vi "0816147.vi"() -> ()   [LabVIEW 2021]
uses:
  <vilib>/gmath/NI_Gmath.lvlib
panel:
  in  "OFF以外的按鍵":T1
  out "七段顯示器小數點":bool
  out "七段顯示器是+ or -":string
  out "七段顯示器":u16[](array[ring])
  out "七段顯示器的=":string
  out "y value 2":dbl format="%.2f"
  in  "formula":string
  out "目前時間":timestamp format="%<%X\n%x>T"
  out "計算機已執行時間":string
  in  "off":bool
  out "算式顯示":string caption="String"
  out "答案":dbl
  in  "計算機背景圖片":u16(ring)
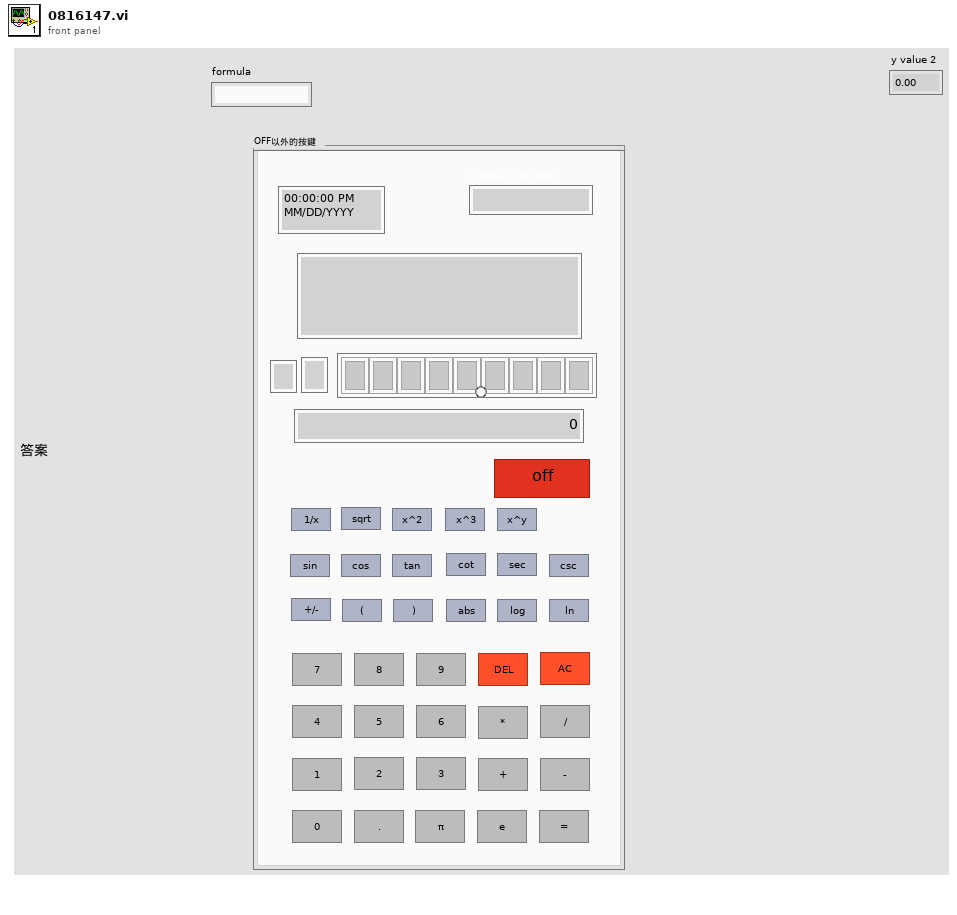
[diagram p1: front panel]
types:
  T1 = cluster{"0":bool, "1":bool, "2":bool, "3":bool, "4":bool, "5":bool, "6":bool, "7":bool, "8":bool, "9":bool, ".":bool, "pi":bool, "e":bool, "/":bool, "*":bool, "-":bool, "=":bool, "DEL":bool, "+":bool, "cos":bool, "sin":bool, "(":bool, ")":bool, "tan":bool, "log":bool, "ln":bool, "x^2":bool, "sqrt":bool, "x^3":bool, "AC":bool, "+/-":bool, "x^y":bool, "csc":bool, "sec":bool, "cot":bool, "1/x":bool, "abs":bool}
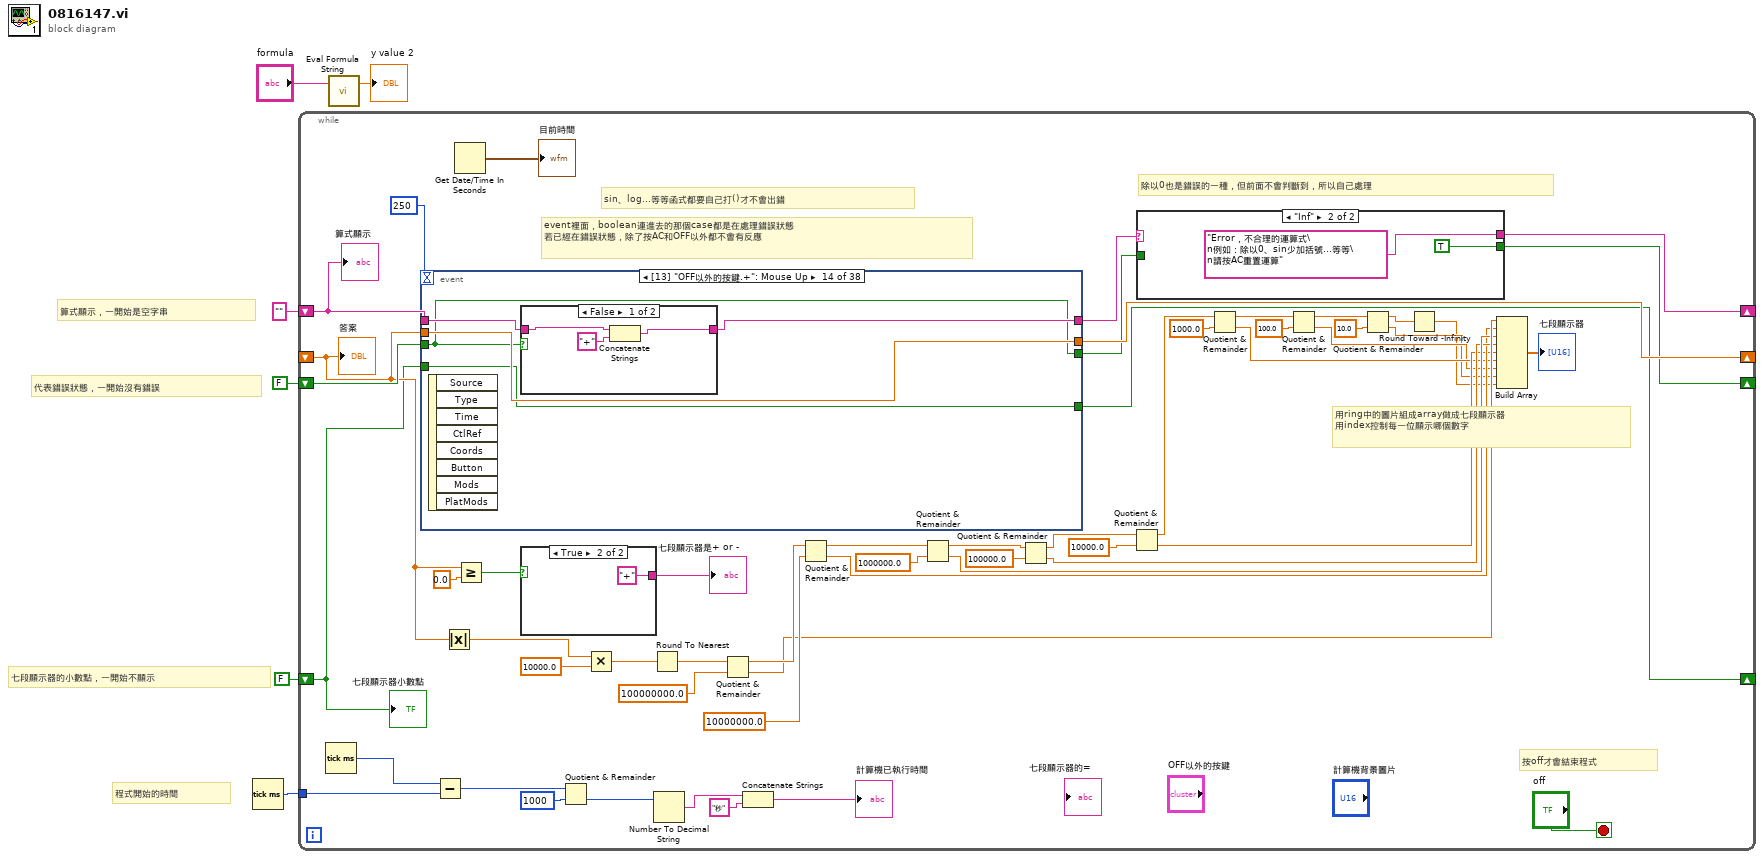
[diagram p0: block diagram]
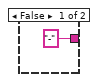
[diagram p2: hidden frame]
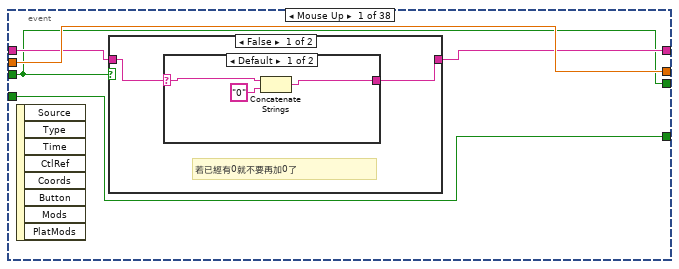
[diagram p4: hidden frame]
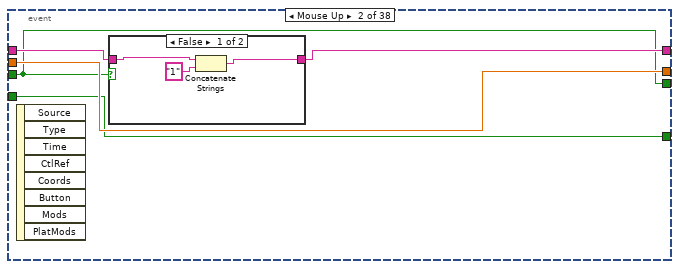
[diagram p7: hidden frame]
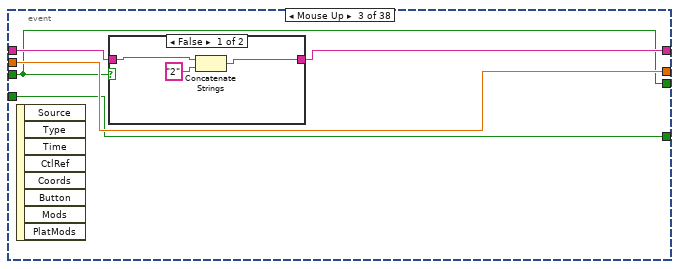
[diagram p9: hidden frame]
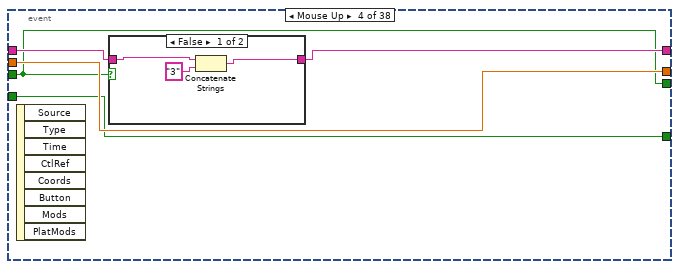
[diagram p11: hidden frame]
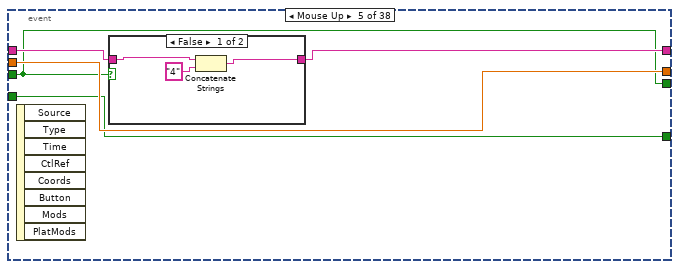
[diagram p13: hidden frame]
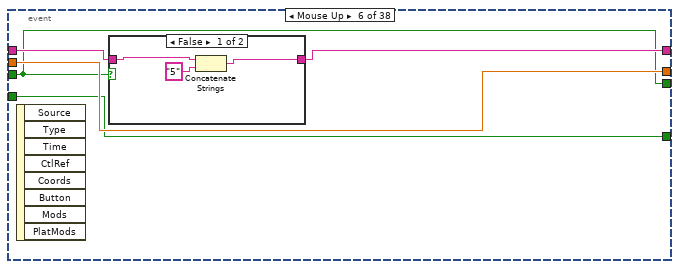
[diagram p15: hidden frame]
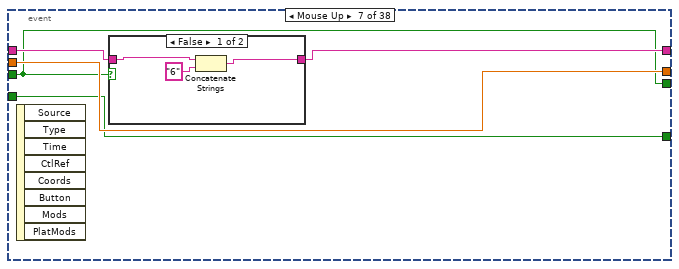
[diagram p17: hidden frame]
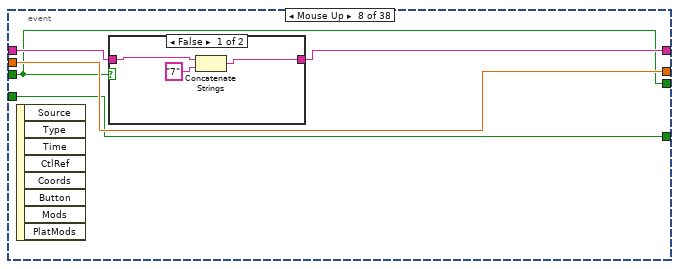
[diagram p19: hidden frame]
diagram:
  # "程式開始的時間"
  # "七段顯示器的小數點，一開始不顯示"
  # "代表錯誤狀態，一開始沒有錯誤"
  # "算式顯示，一開始是空字串"
  n1 = Tick Count (ms)() -> (millisecond timer value=w5:u32)
  n2 = while {
    shift-right: [w44] -> _
    shift-left: "" -> [w43]
    tunnel: w5 -> [w58]
    shift-right: [w50] -> _
    shift-left: _ -> [w39]
    shift-right: [w45] -> _
    shift-left: FALSE -> [w48]
    shift-right: [w20] -> _
    shift-left: FALSE -> [w19]
    stop <- "off" stop-if-true
    # "sin、log...等等函式都要自己打()才不會出錯"
    # "按off才會結束程式"
    # "除以0也是錯誤的一種，但前面不會判斷到，所以自己處理"
    # "用ring中的圖片組成array做成七段顯示器\n用index控制每一位顯示哪個數字"
    # "event裡面，boolean連進去的那個case都是在處理錯誤狀態\n若已經在錯誤狀態，除了按AC和OFF以外都不會有反應"
    n3 = Tick Count (ms)() -> (millisecond timer value=w60:u32)
    n4 = event shown="[13] \"OFF以外的按鍵.+\": Mouse Up" {
      selector: _ -> [_ _ _ _ _ _ _ _ _ _ _ _ _ _ _ _ _ _ _ _ _ _ _ _ _ _ _ _ _ _ _ _ _ _ _ _ _ _]
      dyn-events: _ -> [_ _ _ _ _ _ _ _ _ _ _ _ _ _ _ _ _ _ _ _ _ _ _ _ _ _ _ _ _ _ _ _ _ _ _ _ _ _]
      timeout: 250 -> [_ _ _ _ _ _ _ _ _ _ _ _ _ _ _ _ _ _ _ _ _ _ _ _ _ _ _ _ _ _ _ _ _ _ _ _ _ _]
      tunnel: w43 -> [w70 w82 w91 w100 w109 w118 w127 w136 w144 w153 w162 w172 w183 w197 w206 w215 w224 w230 w247 w264 w273 w282 w291 w300 w309 w319 w328 w336 w345 w354 w363 w372 w382 w389 w400 w408 w417 w432]
      tunnel: [w69 w81 w90 w99 w108 w117 w126 w135 w143 w152 w161 w171 w182 w196 w205 w214 w223 w236 w246 w263 w272 w281 w290 w299 w308 w318 w327 w335 w344 w353 w362 w371 w381 w388 w397 w407 w422 w432] -> w47
      tunnel: [w71 w83 w92 w101 w110 w119 w128 w137 w146 w155 w164 w174 w184 w198 w207 w216 w225 w238 w244 w265 w274 w283 w292 w301 w310 w317 w326 w337 w346 w355 w364 w373 w380 w390 w399 w409 w421 w431] -> w50
      tunnel: w39 -> [w71 w83 w92 w101 w110 w119 w128 w137 w146 w155 w164 w174 w184 w198 w207 w216 w225 _ w244 w265 w274 w283 w292 w301 w310 w317 w326 w337 w346 w355 w364 w373 w380 w390 w399 w409 w416 w431]
      tunnel: [w68 w80 w89 w98 w107 w116 w125 w134 w145 w154 w163 w173 w181 w195 w204 w213 w222 w234 w245 w262 w271 w280 w289 w298 w307 w316 w325 w334 w343 w352 w361 w370 w379 w391 w398 w406 w420 w430] -> w46
      tunnel: w48 -> [w68 w80 w89 w98 w107 w116 w125 w134 w145 w154 w163 w173 w181 w195 w204 w213 w222 _ w245 w262 w271 w280 w289 w298 w307 w316 w325 w334 w343 w352 w361 w370 w379 w391 w398 w406 w418 w430]
      tunnel: [w67 w79 w88 w97 w106 w115 w124 w133 w142 w151 w160 w170 w180 w194 w203 w212 w221 w231 w243 w261 w270 w279 w288 w297 w306 w315 w324 w333 w342 w351 w360 w369 w378 w387 w396 w405 w415 w429] -> w20
      tunnel: w19 -> [w67 w79 w88 w97 w106 w115 w124 w133 w142 w151 w160 w170 w180 w194 w203 w212 w221 _ w243 w261 w270 w279 w288 w297 w306 w315 w324 w333 w342 w351 w360 w369 w378 w387 w396 w405 w415 w429]
      event "OFF以外的按鍵.0": Mouse Up {
        n5 = event-data() -> ()  [unwired: 1 in, 8 out]
        n6 = case shown="False" w68 {
          tunnel: w70 -> [w73 w78]
          tunnel: [w72 w78] -> w69
          frame False {
            # "若已經有0就不要再加0了"
            n7 = case shown="Default" w73 {
              selector: w73 -> [w75 w77]
              tunnel: [w74 w77] -> w72
              frame Default {
                n8 = Concatenate Strings(w75, "0") -> (w74:string)
              }
              frame "0" {
              }
            }
          }
          frame True {
          }
        }
      }
      event "OFF以外的按鍵.1": Mouse Up {
        n9 = event-data() -> ()  [unwired: 1 in, 8 out]
        n10 = case shown="False" w80 {
          tunnel: w82 -> [w86 w87]
          tunnel: [w84 w87] -> w81
          frame False {
            n11 = Concatenate Strings(w86, "1") -> (w84:string)
          }
          frame True {
          }
        }
      }
      event "OFF以外的按鍵.2": Mouse Up {
        n12 = event-data() -> ()  [unwired: 1 in, 8 out]
        n13 = case shown="False" w89 {
          tunnel: w91 -> [w95 w96]
          tunnel: [w93 w96] -> w90
          frame False {
            n14 = Concatenate Strings(w95, "2") -> (w93:string)
          }
          frame True {
          }
        }
      }
      event "OFF以外的按鍵.3": Mouse Up {
        n15 = event-data() -> ()  [unwired: 1 in, 8 out]
        n16 = case shown="False" w98 {
          tunnel: w100 -> [w104 w105]
          tunnel: [w102 w105] -> w99
          frame False {
            n17 = Concatenate Strings(w104, "3") -> (w102:string)
          }
          frame True {
          }
        }
      }
      event "OFF以外的按鍵.4": Mouse Up {
        n18 = event-data() -> ()  [unwired: 1 in, 8 out]
        n19 = case shown="False" w107 {
          tunnel: w109 -> [w113 w114]
          tunnel: [w111 w114] -> w108
          frame False {
            n20 = Concatenate Strings(w113, "4") -> (w111:string)
          }
          frame True {
          }
        }
      }
      event "OFF以外的按鍵.5": Mouse Up {
        n21 = event-data() -> ()  [unwired: 1 in, 8 out]
        n22 = case shown="False" w116 {
          tunnel: w118 -> [w122 w123]
          tunnel: [w120 w123] -> w117
          frame False {
            n23 = Concatenate Strings(w122, "5") -> (w120:string)
          }
          frame True {
          }
        }
      }
      event "OFF以外的按鍵.6": Mouse Up {
        n24 = event-data() -> ()  [unwired: 1 in, 8 out]
        n25 = case shown="False" w125 {
          tunnel: w127 -> [w131 w132]
          tunnel: [w129 w132] -> w126
          frame False {
            n26 = Concatenate Strings(w131, "6") -> (w129:string)
          }
          frame True {
          }
        }
      }
      event "OFF以外的按鍵.7": Mouse Up {
        n27 = event-data() -> ()  [unwired: 1 in, 8 out]
        n28 = case shown="False" w134 {
          tunnel: w136 -> [w140 w141]
          tunnel: [w138 w141] -> w135
          frame False {
            n29 = Concatenate Strings(w140, "7") -> (w138:string)
          }
          frame True {
          }
        }
      }
      event "OFF以外的按鍵.8": Mouse Up {
        n30 = event-data() -> ()  [unwired: 1 in, 8 out]
        n31 = case shown="False" w145 {
          tunnel: w144 -> [w149 w150]
          tunnel: [w147 w150] -> w143
          frame False {
            n32 = Concatenate Strings(w149, "8") -> (w147:string)
          }
          frame True {
          }
        }
      }
      event "OFF以外的按鍵.9": Mouse Up {
        n33 = event-data() -> ()  [unwired: 1 in, 8 out]
        n34 = case shown="False" w154 {
          tunnel: w153 -> [w158 w159]
          tunnel: [w156 w159] -> w152
          frame False {
            n35 = Concatenate Strings(w158, "9") -> (w156:string)
          }
          frame True {
          }
        }
      }
      event "OFF以外的按鍵.pi": Mouse Up {
        # "pi用3.141593代表"
        n36 = event-data() -> ()  [unwired: 1 in, 8 out]
        n37 = case shown="False" w163 {
          tunnel: w162 -> [w166 w169]
          tunnel: [w165 w169] -> w161
          frame False {
            n38 = Number To Fractional String(number=3.141592653589793) -> (F-format string=w167:string)  [unwired: 3 in]
            n39 = Concatenate Strings(w166, w167) -> (w165:string)
          }
          frame True {
          }
        }
      }
      event "OFF以外的按鍵.e": Mouse Up {
        # "e用2.718282代表"
        n40 = event-data() -> ()  [unwired: 1 in, 8 out]
        n41 = case shown="False" w173 {
          tunnel: w172 -> [w176 w179]
          tunnel: [w175 w179] -> w171
          frame False {
            n42 = Number To Fractional String(number=2.718281828459045) -> (F-format string=w177:string)  [unwired: 3 in]
            n43 = Concatenate Strings(w176, w177) -> (w175:string)
          }
          frame True {
          }
        }
      }
      event "OFF以外的按鍵..": Mouse Up {
        # "已有小數點就不再加小數點"
        n44 = event-data() -> ()  [unwired: 1 in, 8 out]
        n45 = case shown="False" w181 {
          tunnel: w183 -> [w186 w193]
          tunnel: [w185 w193] -> w182
          frame False {
            n46 = Match Pattern(string=w186, regular expression="\\.") -> (offset past match=w188:i32)  [unwired: 1 in, 3 out]
            n47 = case shown="0, Default" w188 {
              tunnel: w186 -> [w189 w191]
              tunnel: [w189 w190] -> w185
              frame 0, Default {
              }
              frame -1 {
                n48 = Concatenate Strings(w191, ".") -> (w190:string)
              }
            }
          }
          frame True {
          }
        }
      }
      event "OFF以外的按鍵.+": Mouse Up {
        n49 = event-data() -> ()  [unwired: 1 in, 8 out]
        n50 = case shown="False" w195 {
          tunnel: w197 -> [w201 w202]
          tunnel: [w199 w202] -> w196
          frame False {
            n51 = Concatenate Strings(w201, "+") -> (w199:string)
          }
          frame True {
          }
        }
      }
      event "OFF以外的按鍵.-": Mouse Up {
        n52 = event-data() -> ()  [unwired: 1 in, 8 out]
        n53 = case shown="False" w204 {
          tunnel: w206 -> [w210 w211]
          tunnel: [w208 w211] -> w205
          frame False {
            n54 = Concatenate Strings(w210, "-") -> (w208:string)
          }
          frame True {
          }
        }
      }
      event "OFF以外的按鍵.*": Mouse Up {
        n55 = event-data() -> ()  [unwired: 1 in, 8 out]
        n56 = case shown="False" w213 {
          tunnel: w215 -> [w219 w220]
          tunnel: [w217 w220] -> w214
          frame False {
            n57 = Concatenate Strings(w219, "*") -> (w217:string)
          }
          frame True {
          }
        }
      }
      event "OFF以外的按鍵./": Mouse Up {
        n58 = event-data() -> ()  [unwired: 1 in, 8 out]
        n59 = case shown="False" w222 {
          tunnel: w224 -> [w228 w229]
          tunnel: [w226 w229] -> w223
          frame False {
            n60 = Concatenate Strings(w228, "/") -> (w226:string)
          }
          frame True {
          }
        }
      }
      event "OFF以外的按鍵.=": Mouse Up {
        # "計算結果並確認運算式是否有錯誤"
        n61 = event-data() -> ()  [unwired: 1 in, 8 out]
        n62 = call <vilib>:"Eval Formula String.vi"("formula"=w230) -> ("error out"=w237:errorcluster, "y value"=w238:dbl)  [unwired: 1 in]
        n63 = Match Pattern(string=w230, regular expression="\\.") -> (offset past match=w233:i32)  [unwired: 1 in, 3 out]
        n64 = Unbundle(w237) -> ("status"=w234:bool)  [unwired: 2 out]
        n65 = Number To Fractional String(number=w238) -> (F-format string=w235:string)  [unwired: 3 in]
        n66 = case shown="True" w234 {
          tunnel: [w241 "Error，不合理的運算式\n例如：除以0、sin少加括號...等等\n請按AC重置運算"] -> w236
          tunnel: w235 -> [w241 _]
          frame False {
          }
          frame True {
          }
        }
        n67 = case shown="0, Default" w233 {
          tunnel: [TRUE FALSE] -> w231
          frame 0, Default {
          }
          frame -1 {
          }
        }
      }
      event "OFF以外的按鍵.+/-": Mouse Up {
        # "判斷現在是+或-然後改成另一個"
        n68 = event-data() -> ()  [unwired: 1 in, 8 out]
        n69 = case shown="False" w245 {
          tunnel: w247 -> [w248 w250]
          tunnel: [w248 w249] -> w246
          frame True {
          }
          frame False {
            n70 = String Subset(string=w250, length (rest)=1 ("length (rest)")) -> (substring=w251:string)  [unwired: 1 in]
            n71 = case shown="\"+\", Default" w251 {
              tunnel: w250 -> [w254 w259]
              tunnel: [w253 w256] -> w249
              frame "+", Default {
                n72 = Concatenate Strings("-" ("string"), w254) -> (w253:string)
              }
              frame "-" {
                n73 = String Length(string=w259) -> (length=w258:i32)
                n74 = Decrement(x=w258) -> (x-1=w257:i32)
                n75 = String Subset(string=w259, offset (0)=1, length (rest)=w257) -> (substring=w256:string)
              }
            }
          }
        }
      }
      event "OFF以外的按鍵.(": Mouse Up {
        n76 = event-data() -> ()  [unwired: 1 in, 8 out]
        n77 = case shown="False" w262 {
          tunnel: w264 -> [w268 w269]
          tunnel: [w266 w269] -> w263
          frame False {
            n78 = Concatenate Strings(w268, "(") -> (w266:string)
          }
          frame True {
          }
        }
      }
      event "OFF以外的按鍵.)": Mouse Up {
        n79 = event-data() -> ()  [unwired: 1 in, 8 out]
        n80 = case shown="False" w271 {
          tunnel: w273 -> [w277 w278]
          tunnel: [w275 w278] -> w272
          frame False {
            n81 = Concatenate Strings(w277, ")") -> (w275:string)
          }
          frame True {
          }
        }
      }
      event "OFF以外的按鍵.sin": Mouse Up {
        n82 = event-data() -> ()  [unwired: 1 in, 8 out]
        n83 = case shown="False" w280 {
          tunnel: w282 -> [w286 w287]
          tunnel: [w284 w287] -> w281
          frame False {
            n84 = Concatenate Strings(w286, "sin") -> (w284:string)
          }
          frame True {
          }
        }
      }
      event "OFF以外的按鍵.cos": Mouse Up {
        n85 = event-data() -> ()  [unwired: 1 in, 8 out]
        n86 = case shown="False" w289 {
          tunnel: w291 -> [w295 w296]
          tunnel: [w293 w296] -> w290
          frame False {
            n87 = Concatenate Strings(w295, "cos") -> (w293:string)
          }
          frame True {
          }
        }
      }
      event "OFF以外的按鍵.tan": Mouse Up {
        n88 = event-data() -> ()  [unwired: 1 in, 8 out]
        n89 = case shown="False" w298 {
          tunnel: w300 -> [w304 w305]
          tunnel: [w302 w305] -> w299
          frame False {
            n90 = Concatenate Strings(w304, "tan") -> (w302:string)
          }
          frame True {
          }
        }
      }
      event "OFF以外的按鍵.cot": Mouse Up {
        n91 = event-data() -> ()  [unwired: 1 in, 8 out]
        n92 = case shown="False" w307 {
          tunnel: w309 -> [w312 w314]
          tunnel: [w311 w314] -> w308
          frame False {
            n93 = Concatenate Strings(w312, "cot") -> (w311:string)
          }
          frame True {
          }
        }
      }
      event "OFF以外的按鍵.sec": Mouse Up {
        n94 = event-data() -> ()  [unwired: 1 in, 8 out]
        n95 = case shown="False" w316 {
          tunnel: w319 -> [w321 w323]
          tunnel: [w320 w323] -> w318
          frame False {
            n96 = Concatenate Strings(w321, "sec") -> (w320:string)
          }
          frame True {
          }
        }
      }
      event "OFF以外的按鍵.csc": Mouse Up {
        n97 = event-data() -> ()  [unwired: 1 in, 8 out]
        n98 = case shown="False" w325 {
          tunnel: w328 -> [w330 w332]
          tunnel: [w329 w332] -> w327
          frame False {
            n99 = Concatenate Strings(w330, "csc") -> (w329:string)
          }
          frame True {
          }
        }
      }
      event "OFF以外的按鍵.log": Mouse Up {
        n100 = event-data() -> ()  [unwired: 1 in, 8 out]
        n101 = case shown="False" w334 {
          tunnel: w336 -> [w340 w341]
          tunnel: [w338 w341] -> w335
          frame False {
            n102 = Concatenate Strings(w340, "log") -> (w338:string)
          }
          frame True {
          }
        }
      }
      event "OFF以外的按鍵.ln": Mouse Up {
        n103 = event-data() -> ()  [unwired: 1 in, 8 out]
        n104 = case shown="False" w343 {
          tunnel: w345 -> [w349 w350]
          tunnel: [w347 w350] -> w344
          frame False {
            n105 = Concatenate Strings(w349, "ln") -> (w347:string)
          }
          frame True {
          }
        }
      }
      event "OFF以外的按鍵.sqrt": Mouse Up {
        n106 = event-data() -> ()  [unwired: 1 in, 8 out]
        n107 = case shown="False" w352 {
          tunnel: w354 -> [w358 w359]
          tunnel: [w356 w359] -> w353
          frame False {
            n108 = Concatenate Strings(w358, "sqrt") -> (w356:string)
          }
          frame True {
          }
        }
      }
      event "OFF以外的按鍵.x^2": Mouse Up {
        n109 = event-data() -> ()  [unwired: 1 in, 8 out]
        n110 = case shown="False" w361 {
          tunnel: w363 -> [w367 w368]
          tunnel: [w365 w368] -> w362
          frame False {
            n111 = Concatenate Strings(w367, "^2") -> (w365:string)
          }
          frame True {
          }
        }
      }
      event "OFF以外的按鍵.x^3": Mouse Up {
        n112 = event-data() -> ()  [unwired: 1 in, 8 out]
        n113 = case shown="False" w370 {
          tunnel: w372 -> [w376 w377]
          tunnel: [w374 w377] -> w371
          frame False {
            n114 = Concatenate Strings(w376, "^3") -> (w374:string)
          }
          frame True {
          }
        }
      }
      event "OFF以外的按鍵.x^y": Mouse Up {
        n115 = event-data() -> ()  [unwired: 1 in, 8 out]
        n116 = case shown="False" w379 {
          tunnel: w382 -> [w384 w386]
          tunnel: [w383 w386] -> w381
          frame False {
            n117 = Concatenate Strings(w384, "^") -> (w383:string)
          }
          frame True {
          }
        }
      }
      event "OFF以外的按鍵.1/x": Mouse Up {
        n118 = event-data() -> ()  [unwired: 1 in, 8 out]
        n119 = case shown="False" w391 {
          tunnel: w389 -> [w394 w395]
          tunnel: [w392 w395] -> w388
          frame False {
            n120 = Concatenate Strings(w394, "^(-1)" ("string")) -> (w392:string)
          }
          frame True {
          }
        }
      }
      event "OFF以外的按鍵.abs": Mouse Up {
        n121 = event-data() -> ()  [unwired: 1 in, 8 out]
        n122 = case shown="False" w398 {
          tunnel: w400 -> [w402 w404]
          tunnel: [w401 w404] -> w397
          frame False {
            n123 = Concatenate Strings(w402, "abs") -> (w401:string)
          }
          frame True {
          }
        }
      }
      event "OFF以外的按鍵.DEL": Mouse Up {
        # "刪掉最右邊的字元"
        n124 = event-data() -> ()  [unwired: 1 in, 8 out]
        n125 = case shown="False" w406 {
          tunnel: w408 -> [w411 w414]
          tunnel: [w410 w414] -> w407
          frame False {
            n126 = String Length(string=w411) -> (length=w412:i32)
            n127 = Decrement(x=w412) -> (x-1=w413:i32)
            n128 = String Subset(string=w411, length (rest)=w413) -> (substring=w410:string)  [unwired: 1 in]
          }
          frame True {
          }
        }
      }
      event "OFF以外的按鍵.AC": Mouse Up {
        # "跳出確認提示"
        n129 = event-data() -> ()  [unwired: 1 in, 8 out]
        n130 = call "Display Message to User"() -> ("Yes"=w419:bool)  [unwired: 10 in, 1 out]
        n131 = case shown="True" w419 {
          tunnel: [w424 ""] -> w422
          tunnel: [w423 0.0 ("y value")] -> w421
          tunnel: [w425 FALSE ("status")] -> w420
          tunnel: w418 -> [w425 _]
          tunnel: w417 -> [w424 _]
          tunnel: w416 -> [w423 _]
          frame False {
          }
          frame True {
            # "把所有東西清空"
          }
        }
      }
      event Timeout {
        # "timeout就照原本的樣子"
        n132 = event-data() -> ()  [unwired: 1 in, 3 out]
      }
    }
    n133 = Subtract(x=w60, y=w58) -> (x-y=w59:u32)
    n134 = Absolute Value(x=w39) -> (abs(x)=w8:dbl)
    n135 = Get Date/Time In Seconds() -> (seconds since 1Jan1904=→"目前時間":timestamp)
    n136 = Greater Or Equal?(x=w39, y=0.0) -> (x >= y?=w41:bool)
    n137 = case shown="True" w41 {
      tunnel: ["-" "+"] -> w40
      frame False {
      }
      frame True {
      }
    }
    "七段顯示器是+ or -" <- w40
    n138 = Quotient & Remainder(x=w59, y=u32 1000) -> (floor(x/y)=w56:u32)  [unwired: 1 out]
    n139 = Multiply(x=w8, y=10000.0) -> (x*y=w17:dbl)
    n140 = Round To Nearest(number=w17) -> (nearest integer value=w7:dbl)
    n141 = Number To Decimal String(number=w56) -> (decimal integer string=w55:string)  [unwired: 1 in]
    n142 = Quotient & Remainder(x=w7, y=100000000.0) -> (x-y*floor(x/y)=w34:dbl, floor(x/y)=w31:dbl)
    n143 = Concatenate Strings(w55, "秒" ("string")) -> (→"計算機已執行時間":string)
    n144 = Quotient & Remainder(x=w34, y=10000000.0) -> (x-y*floor(x/y)=w33:dbl, floor(x/y)=w15:dbl)
    n145 = Quotient & Remainder(x=w33, y=1000000.0) -> (x-y*floor(x/y)=w32:dbl, floor(x/y)=w30:dbl)
    n146 = Quotient & Remainder(x=w32, y=100000.0) -> (x-y*floor(x/y)=w16:dbl, floor(x/y)=w29:dbl)
    n147 = Quotient & Remainder(x=w16, y=10000.0) -> (x-y*floor(x/y)=w23:dbl, floor(x/y)=w14:dbl)
    n148 = case shown="\"Inf\"" w47 {
      selector: w47 -> [w63 _]
      tunnel: w46 -> [w64 _]
      tunnel: [w64 TRUE] -> w45
      tunnel: [w63 "Error，不合理的運算式\n例如：除以0、sin少加括號...等等\n請按AC重置運算"] -> w44
      frame "False", Default {
      }
      frame "Inf" {
      }
    }
    n149 = Quotient & Remainder(x=w23, y=1000.0) -> (x-y*floor(x/y)=w22:dbl, floor(x/y)=w13:dbl)
    n150 = Quotient & Remainder(x=w22, y=100.0) -> (x-y*floor(x/y)=w21:dbl, floor(x/y)=w12:dbl)
    n151 = Quotient & Remainder(x=w21, y=10.0) -> (x-y*floor(x/y)=w10:dbl, floor(x/y)=w11:dbl)
    n152 = Round Toward -Infinity(1:w10) -> (0:w9:dbl)
    n153 = Build Array(w31, w15, w30, w29, w14, w13, w12, w11, w9) -> (→"七段顯示器":dbl[])
    "算式顯示" <- w43
    "答案" <- w39
    "七段顯示器小數點" <- w19
  }
  n154 = call <vilib>:"Eval Formula String.vi"("formula"="formula") -> ("y value"=→"y value 2":dbl)  [unwired: 1 in, 1 out]
